vi "PP.PNG.File.Decode.vi"(5 "Password":string, 7 "error in":errorcluster, 9 "File Folder Out":path, 10 "PNG In":path) -> (0 "error out":errorcluster)   [LabVIEW 2020, in "PixPack.lvlib"]
uses:
  PixPack.lvlib
  b03004ab-3047-4f95-8fc8-d41fbc51de86.vi
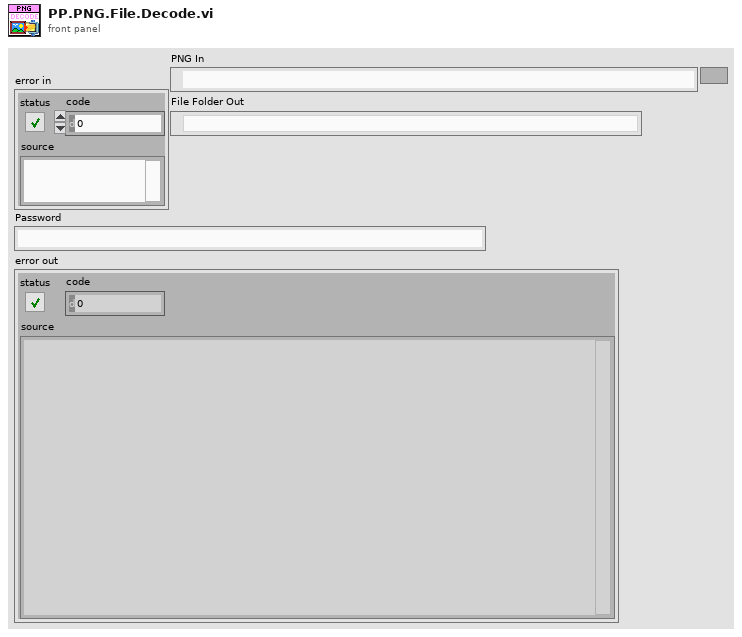
[diagram p1: front panel]
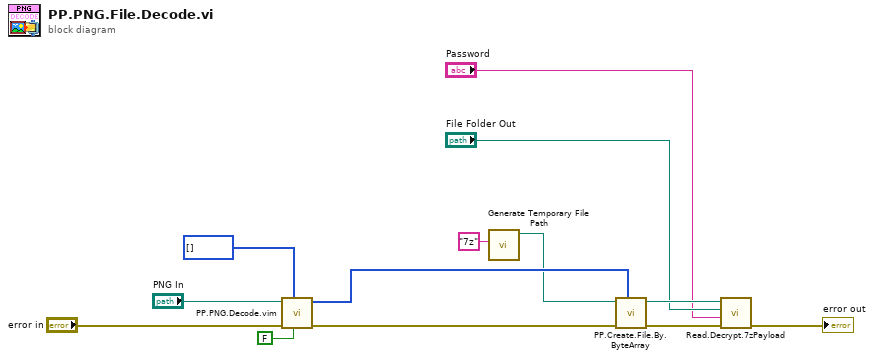
[diagram p0: block diagram]
diagram:
  n1 = call "PP.PNG.Decode.vim"("Get Image Data (F)"=FALSE, "Data Type (Default)"=u8[] [] ("data"), "error in"="error in", "PNG In"="PNG In") -> ("error out"=w12:errorcluster, "Value"=w10:u8[])  [unwired: 3 in, 3 out]
  n2 = call <vilib>:"Generate Temporary File Path.vi"("Temporary File Extension (tmp)"="7z") -> ("Unique Temporary File Path"=w6:path)  [unwired: 9 in, 1 out]
  n3 = call "PP.Create.File.By.ByteArray.vi"("u8 Data[]"=w10, "error in"=w12, "file path (use dialog)"=w6) -> ("error out"=w9:errorcluster, "file path out"=w7:path)  [unwired: 7 in]
  n4 = call "Read.Decrypt.7zPayload.vi"("error in (no error)"=w9, "Password"="Password", "File Folder Out"="File Folder Out", "File Path"=w7) -> ("error out"=→"error out":errorcluster)  [unwired: 7 in]
